vi "Write Servo Switch.vi"(8 "error in (no error)":errorcluster, 10 "Servo Switch":refnum<class "Servo Switch.lvclass">, 11 "tCRD in":refnum<class "Aircraft OPCCRD.lvclass">) -> (0 "error out":errorcluster, 3 "tCRD out":refnum<class "Aircraft OPCCRD.lvclass">)   [LabVIEW 2015]
uses:
  Aircraft OPCCRD.lvclass
  Switch/Servo Switch.lvclass
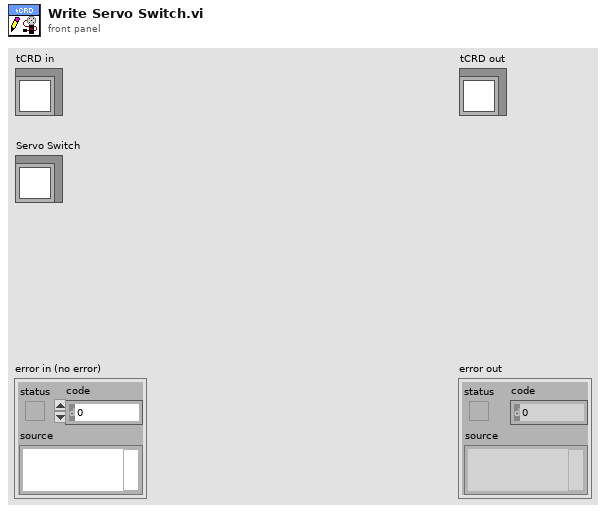
[diagram p1: front panel]
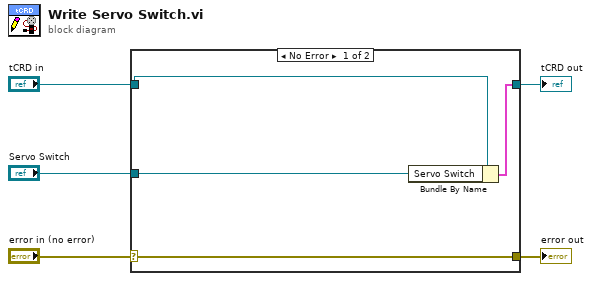
[diagram p0: block diagram]
diagram:
  n1 = case shown="No Error" "error in (no error)" {
    selector: "error in (no error)" -> [w9 w10]
    tunnel: [w9 w10] -> w4
    tunnel: [w7 w11] -> w2
    tunnel: "tCRD in" -> [w8 w11]
    tunnel: "Servo Switch" -> [w6 _]
    frame No Error {
      n2 = Bundle By Name(cluster=w8, "Servo Switch"=w6) -> (w7:cluster{})
    }
    frame Error {
    }
  }
  "error out" <- w4
  "tCRD out" <- w2
